vi "XY Graph Check-Uncheck Menu Items.vi"(8 "Error In":errorcluster, 9 "Coords":T2, 10 "Menu in":refnum<k9>, 11 "XY Graph Refnum":T3) -> (0 "Error Out (dup)":errorcluster, 1 "Click Location":T1)   [LabVIEW 2019, in "XY Graph Add-Ons.lvlib"]
uses:
  XY Graph Add-Ons.lvlib
  XY Graph Refnum.ctl
  <vilib>/Utility/miscctls.llb/LVPoint32TypeDef.ctl
  XY Graph Click Location.ctl
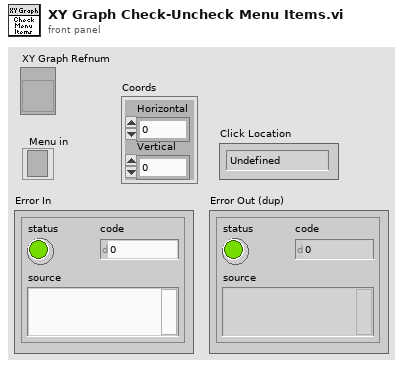
[diagram p1: front panel]
types:
  T1 = typedef "XY Graph Click Location.ctl" = enum16{"Undefined", "Plot Area", "Plot Legend", "Scale Legend", "Graph Palette", "Cursor Legend", "Graph Border"}
  T2 = typedef "LVPoint32TypeDef.ctl" = cluster{"Horizontal":i32, "Vertical":i32}
  T3 = typedef "XY Graph Add-Ons.lvlib/XY Graph Refnum.ctl" = refnum<vi>
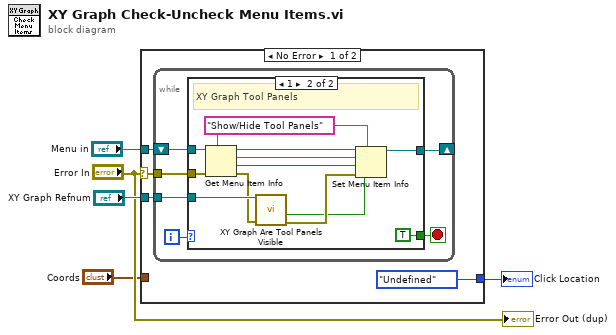
[diagram p0: block diagram]
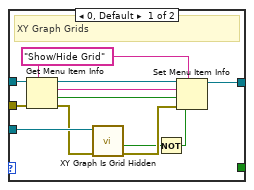
[diagram p2: hidden frame]
diagram:
  n1 = case shown="No Error" "Error In" {
    selector: "Error In" -> [w8 _]
    tunnel: "XY Graph Refnum" -> [w7 _]
    tunnel: "Menu in" -> [w9 _]
    tunnel: "Coords" -> [_ _]
    tunnel: [XY_Graph_Click_Location."Undefined" ("Click Location") _] -> w1
    frame No Error {
      n2 = while {
        tunnel: w7 -> [w15]
        tunnel: w8 -> [w12]
        shift-right: [w11] -> _
        shift-left: w9 -> [w14]
        i -> [w13]
        stop <- w10 stop-if-true
        n3 = case shown="1" w13 {
          tunnel: w15 -> [w27 w32]
          tunnel: w14 -> [w26 w39]
          tunnel: w12 -> [w24 w38]
          tunnel: [w16 w33] -> w11
          tunnel: [_ TRUE] -> w10
          frame 0, Default {
            w17 = "Show/Hide Grid" ("item tag")
            # "XY Graph Grids"
            n4 = Get Menu Item Info(7:w17, 8:w24, 11:w26) -> (0:w25:errorcluster, 1:w19:bool, 2:w18:string, 3:w23:refnum<k9>)  [unwired: 3 out]
            n5 = call "XY Graph Is Grid Hidden.vi"("Error In"=w25, "XY Graph Ref"=w27) -> ("Error Out (dup)"=w22:errorcluster, "Hidden Grid(s)"=w21:bool)  [unwired: 8 in]
            n6 = Not(x=w21) -> (.not. x?=w20:bool)
            n7 = Set Menu Item Info(6:w20, 7:w17, 8:w22, 9:w19, 10:w18, 11:w23) -> (3:w16:refnum<k9>)  [unwired: 1 in, 1 out]
          }
          frame 1 {
            w34 = "Show/Hide Tool Panels" ("item tag")
            # "XY Graph Tool Panels"
            n8 = Get Menu Item Info(7:w34, 8:w38, 11:w39) -> (0:w31:errorcluster, 1:w36:bool, 2:w35:string, 3:w37:refnum<k9>)  [unwired: 3 out]
            n9 = call "XY Graph Are Tool Panels Visible.vi"("Error In"=w31, "XY Graph Ref"=w32) -> ("Error Out"=w30:errorcluster, "Any Panel Visible?"=w29:bool)  [unwired: 7 in, 1 out]
            n10 = Set Menu Item Info(6:w29, 7:w34, 8:w30, 9:w36, 10:w35, 11:w37) -> (3:w33:refnum<k9>)  [unwired: 1 in, 1 out]
          }
        }
      }
    }
    frame Error {
    }
  }
  "Click Location" <- w1
  "Error Out (dup)" <- "Error In"
